vi "Create File.vi"(8 "error in":errorcluster, 11 "Root Path":path) -> (0 "error out":errorcluster, 1 "File Path Out":path, 3 "Refnum Out":refnum<file>)   [LabVIEW 2021]
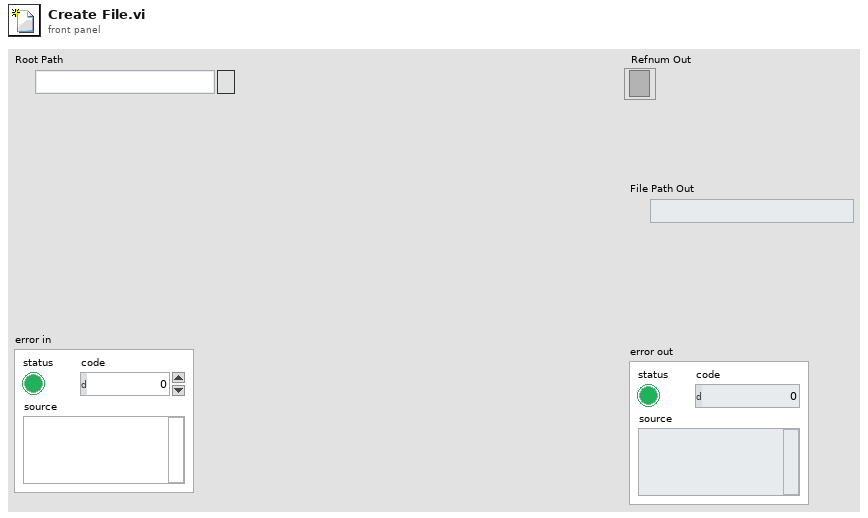
[diagram p1: front panel]
types:
  T1 = enum16{"open", "replace", "create", "open or create", "replace or create", "replace or create with confirmation"}
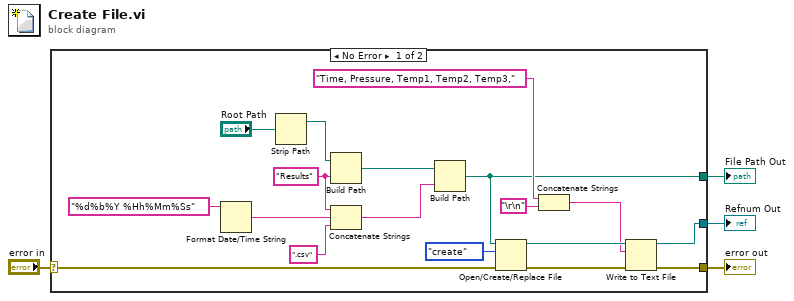
[diagram p0: block diagram]
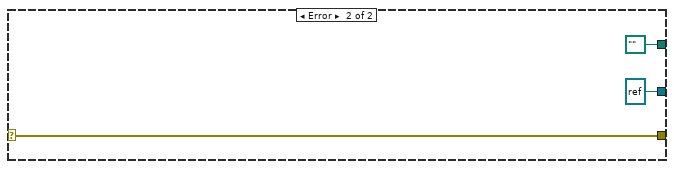
[diagram p2: hidden frame]
diagram:
  n1 = case shown="No Error" "error in" {
    selector: "error in" -> [w14 w25]
    tunnel: [w10 w25] -> w3
    tunnel: [w6 refnum<file> refnum ("refnum out")] -> w2
    tunnel: [w5 path "" ("appended path")] -> w1
    frame No Error {
      w17 = "Results" ("string")
      n2 = Format Date/Time String(time format string (%c)="%d%b%Y %Hh%Mm%Ss") -> (date/time string=w21:string)  [unwired: 2 in]
      n3 = Strip Path(path="Root Path") -> (stripped path=w18:path)  [unwired: 1 out]
      n4 = Build Path(base path=w18, name or relative path=w17) -> (appended path=w16:path)
      n5 = Concatenate Strings "Concatenate Strings"(w17, w21, ".csv" ("string")) -> (w15:string)
      n6 = Build Path(base path=w16, name or relative path=w15) -> (appended path=w5:path)
      n7 = Open/Create/Replace File(file path (use dialog)=w5, error in=w14, operation (0:open)=T1."create") -> (refnum out=w12:refnum<file>, error out=w11:errorcluster)  [unwired: 3 in, 1 out]
      n8 = Concatenate Strings "Concatenate Strings"("Time, Pressure, Temp1, Temp2, Temp3," ("string"), "\r\n") -> (w7:string)
      n9 = Write to Text File(file (use dialog)=w12, text=w7, error in=w11) -> (refnum out=w6:refnum<file>, error out=w10:errorcluster)  [unwired: 1 in, 1 out]
    }
    frame Error {
    }
  }
  "error out" <- w3
  "File Path Out" <- w1
  "Refnum Out" <- w2
